vi "WavePolarizatorGui.vi"(1 "error out 2":errorcluster, 2 "Polarisatior":enum16{"Radial", "Azimuthal"}(ring)) -> (0 "error out":errorcluster)   [LabVIEW 2011]
uses:
  C:/Entwicklungsdaten/Aktuell/Source/LV Source/arcoptix/LCDriver.dll
  Entwicklungsdaten/Aktuell/Source/LV Source/arcoptix/LCDriver.dll
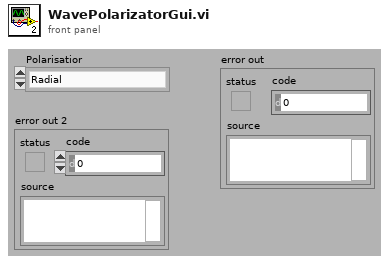
[diagram p1: front panel]
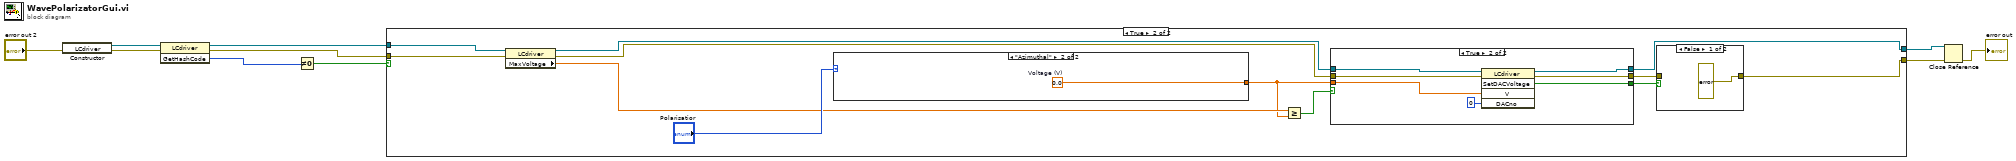
[diagram p0: block diagram]
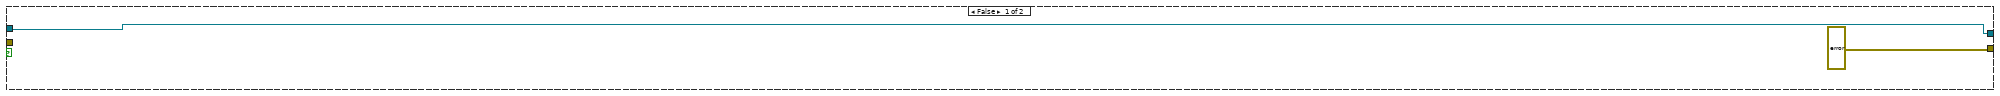
[diagram p2: hidden frame]
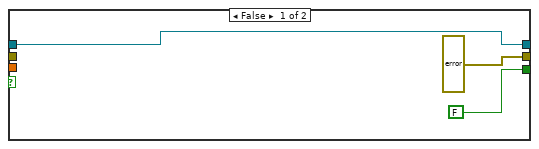
[diagram p4: hidden frame]
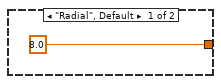
[diagram p5: hidden frame]
diagram:
  n1 = constructor class="LCdriver"(error in="error out 2") -> (reference out=w8:refnum<k24>, error out=w6:errorcluster)  [unwired: 2 in, 1 out]
  n2 = invoke class="LCdriver" method="GetHashCode"(reference=w8, error in=w6) -> (reference out=w7:refnum<k24>, error out=w5:errorcluster, "GetHashCode"=w3:i32)  [unwired: 1 in]
  n3 = Not Equal To 0?(x=w3) -> (x != 0?=w4:bool)
  n4 = case shown="True" w4 {
    tunnel: [errorcluster {"status"=FALSE, "code"=0, "source"="Error Methode ArcOptix"} ("error out") w13] -> w10
    tunnel: [w12 w19] -> w9
    tunnel: w7 -> [w12 w22]
    tunnel: w5 -> [_ w21]
    frame False {
    }
    frame True {
      n5 = property class="LCdriver"(reference=w22, error in=w21) -> (reference out=w24:refnum<k24>, error out=w23:errorcluster, "MaxVoltage"=w18:dbl)
      n6 = case shown="\"Azimuthal\"" "Polarisatior" {
        tunnel: [8.0 ("Voltage (V)") w38] -> w17
        frame "Radial", Default {
        }
        frame "Azimuthal" {
          w38 = 0.0  # Voltage (V)
        }
      }
      n7 = Greater Or Equal?(x=w18, y=w17) -> (x >= y?=w16:bool)
      n8 = case shown="True" w16 {
        tunnel: w24 -> [w29 w35]
        tunnel: w23 -> [_ w34]
        tunnel: [FALSE ("SetDACVoltage") w33] -> w15
        tunnel: [w29 w32] -> w19
        tunnel: [errorcluster {"status"=FALSE, "code"=0, "source"="voltage to high must be under 8,8"} ("error out") w31] -> w14
        tunnel: w17 -> [_ w30]
        frame False {
        }
        frame True {
          n9 = invoke class="LCdriver" method="SetDACVoltage"(reference=w35, error in=w34, "V"=w30, "DACno"=u8 0) -> (reference out=w32:refnum<k24>, error out=w31:errorcluster, "SetDACVoltage"=w33:bool)  [unwired: 1 in, 2 out]
        }
      }
      n10 = case shown="False" w15 {
        tunnel: w14 -> [_ w26]
        tunnel: [errorcluster {"status"=FALSE, "code"=0, "source"="error polarisator value change"} ("error out") w26] -> w13
        frame False {
        }
        frame True {
        }
      }
    }
  }
  n11 = Close Reference(reference=w9, error in (no error)=w10) -> (error out=→"error out":errorcluster)
